vi "SearchJSONArray.vi"(5 "eventinfoJSON":variant, 6 "JSONArray":variant) -> (0 "Boolean":bool)   [LabVIEW 2018]
uses:
  <vilib>/LVH/i3 JSON/JSON Parsing/Get Array Value at Index Files/Get Array Value at Index - Object.vi
  <vilib>/LVH/i3 JSON/JSON Parsing/Get Object Parameter Files/Get Object Parameter - Object.vi
  <vilib>/LVH/i3 JSON/i3-json.lvlib
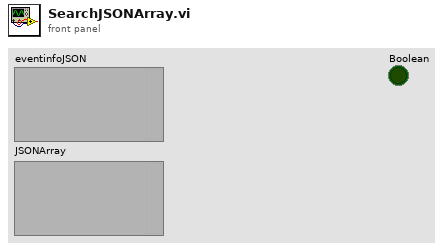
[diagram p1: front panel]
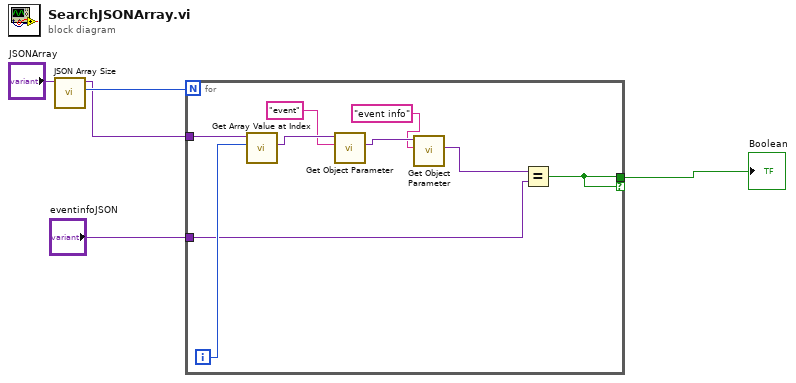
[diagram p0: block diagram]
diagram:
  n1 = call <vilib>:"JSON Array Size.vi"("JSON Tree In (JSON Array)"="JSONArray") -> ("Array Size"=w5:i32, "JSON Tree Passthrough (JSON Array)"=w4:variant)  [unwired: 8 in, 1 out]
  n2 = for {
    N: w5 -> [_]
    tunnel: w4 -> [w14]
    tunnel: "eventinfoJSON" -> [w7]
    tunnel: [w6] -> w1 if=w6
    i -> [w13]
    n3 = call-poly <vilib>:"Get Array Value at Index.vi"("Index"=w13, "JSON Tree In (JSON Array)"=w14) -> ("JSON Object"=w12:variant)  [unwired: 6 in, 3 out]
    n4 = call-poly <vilib>:"Get Object Parameter.vi"("Parameter Name"="event", "JSON Tree In (JSON Object)"=w12) -> ("JSON Object"=w10:variant)  [unwired: 6 in, 3 out]
    n5 = call-poly <vilib>:"Get Object Parameter.vi"("Parameter Name"="event info", "JSON Tree In (JSON Object)"=w10) -> ("JSON Object"=w8:variant)  [unwired: 6 in, 3 out]
    n6 = Equal?(x=w8, y=w7) -> (x = y?=w6:bool)
  }
  "Boolean" <- w1
